vi "multiColorWormSetExposureTimeMultiplier.vi"(1 "exposureTimeMultiplier":dbl, 2 "molecule":string) -> ()   [LabVIEW 2017]
uses:
  globalUtilities.vi
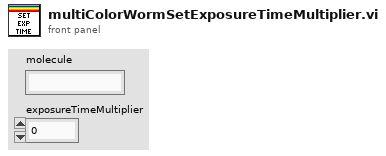
[diagram p1: front panel]
types:
  T1 = cluster{"laserWavelength":dbl, "exposureTime":dbl, "filterWheelPosition":u8, "name":string, "exposureTimeMultiplier":dbl}[]
  T2 = cluster{"laserWavelength":dbl, "exposureTime":dbl, "filterWheelPosition":u8, "name":string, "exposureTimeMultiplier":dbl}
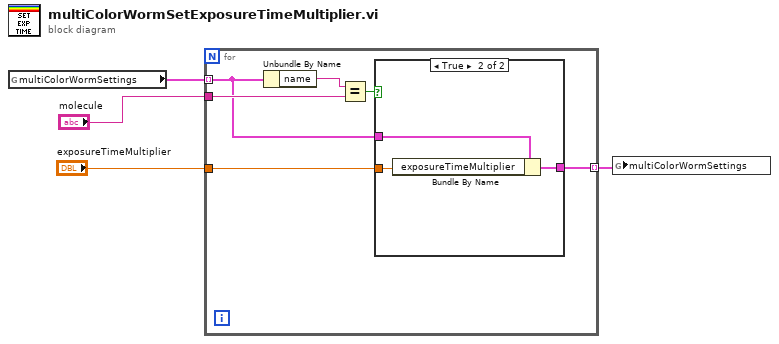
[diagram p0: block diagram]
diagram:
  n1 = global read "globalUtilities.vi" "multiColorWormSettings"() -> (w4:T1)
  n2 = for {
    tunnel: w4 -> [w7] mode=indexing
    tunnel: "molecule" -> [w9]
    tunnel: "exposureTimeMultiplier" -> [w6]
    tunnel: [w5] -> w1 mode=indexing
    n3 = Unbundle By Name(w7) -> ("name"=w10:string)
    n4 = Equal?(x=w10, y=w9) -> (x = y?=w8:bool)
    n5 = case shown="True" w8 {
      tunnel: w7 -> [w11 w14]
      tunnel: w6 -> [_ w13]
      tunnel: [w11 w12] -> w5
      frame False {
      }
      frame True {
        n6 = Bundle By Name(cluster=w14, "exposureTimeMultiplier"=w13) -> (w12:T2)
      }
    }
  }
  n7 = global write "globalUtilities.vi" "multiColorWormSettings"(w1) -> ()
